vi "NILIA_Set_Para.vi"(7 "fs":dbl=50000.0, 10 "rolloff":T1(ring), 11 "TC [sec]":dbl=0.25 format="%.2f") -> (0 "3rd stages":i32, 1 "3rd decimation":i32, 2 "2nd decimation":i32, 3 "1st decimation":i32, 4 "corr":dbl)   [LabVIEW 2012]
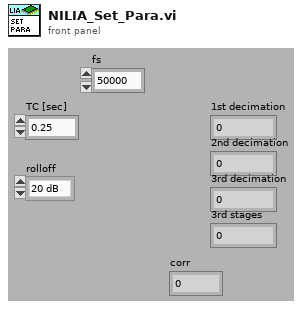
[diagram p1: front panel]
types:
  T1 = enum16{"20 dB", "40 dB", "60 dB", "80 dB", "100 dB", "120 dB", "140 dB", "160 dB", "180 dB", "200 dB"}
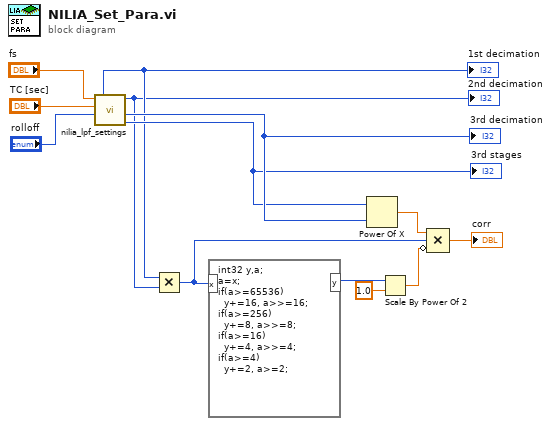
[diagram p0: block diagram]
diagram:
  n1 = call "nilia_lpf_settings.vi"("rolloff"="rolloff", "TC [sec]"="TC [sec]", "fs"="fs") -> ("3rd stages"=w7:i32, "3rd decimation"=w8:i32, "2nd decimation"=w5:i32, "1st decimation"=w6:i32)  [unwired: 1 in, 4 out]
  "1st decimation" <- w6
  "2nd decimation" <- w5
  "3rd decimation" <- w8
  "3rd stages" <- w7
  n2 = Multiply(x=w6, y=w5) -> (x*y=w3:i32)
  n3 = formula code="int32 y,a;\na=x;\nif(a>=65536)\n  y+=16, a>>=16;\nif(a>=256)\n  y+=8, a>>=8;\nif(a>=16)\n  y+=4, a>>=4;\nif(a>=4)\n  y+=2, a>=2;"("x"=w3) -> ("y"=w10:i32)
  n4 = Power Of X(1:w8, 2:w7) -> (0:w4:dbl)
  n5 = Scale By Power Of 2(n=w10, x=1.0) -> (x*2^n=w2:dbl)
  n6 = Compound Arithmetic op=MULTIPLY(w4, w3, invert w2) -> (→"corr":dbl)
